vi "Set Nb_Sample.vi"(8 "error in (no error)":errorcluster caption="entrée d'erreur (pas d'erreur)", 10 "Nb Sample":u16, 11 "Class DIO en entrée":refnum<class "Class Instrument Ana.lvclass">) -> (0 "error out":errorcluster caption="sortie d'erreur", 3 "Class DIO en Sortie":refnum<class "Class Instrument Ana.lvclass">)   [LabVIEW 2020, in "Library Instrument & Equipement.lvlib" / "Library Instruments.lvlib" / "Class Instrument Ana.lvclass"]
uses:
  Class Instrument Ana.lvclass
  Class Instrument Ana.lvclass/Class Instrument Ana.ctl
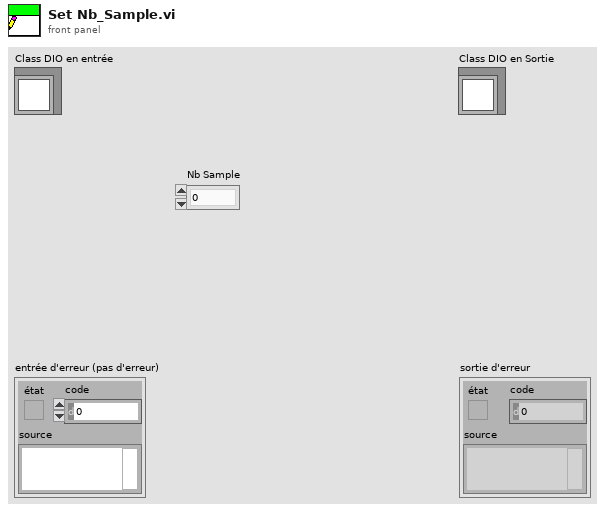
[diagram p1: front panel]
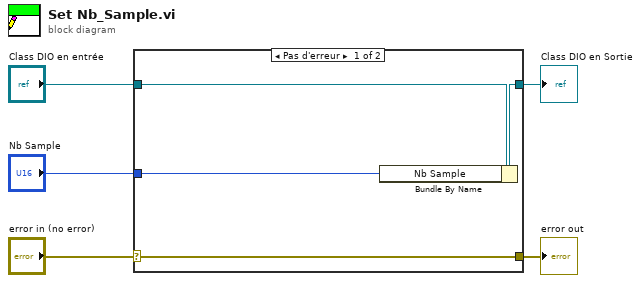
[diagram p0: block diagram]
diagram:
  n1 = case shown="Pas d'erreur" "error in (no error)" {
    selector: "error in (no error)" -> [w9 w10]
    tunnel: [w9 w10] -> w4
    tunnel: [w7 w11] -> w2
    tunnel: "Class DIO en entrée" -> [w8 w11]
    tunnel: "Nb Sample" -> [w6 _]
    frame No Error {
      n2 = Bundle By Name(cluster=w8, "Nb Sample"=w6) -> (w7:refnum<class "Class Instrument Ana.lvclass">)
    }
    frame Error {
    }
  }
  "error out" <- w4
  "Class DIO en Sortie" <- w2
